vi "DIM_DIO.get service names.vi"(0 "i ref in":refnum<vi>, 5 "error in (no error)":errorcluster) -> (14 "i ref out":refnum<vi>, 16 "writeService":string, 17 "readService":string, 19 "error out":errorcluster)   [LabVIEW 2014, in "DIM_DIO.lvlib"]
doc: "Gets the names of DIM services that are connected to the digital input and output. If a services name equals \"N/A\", the service does not exist and is not created/connected.\n\nLicense Agreement for this software:\n\nCopyright (C)\nGesellschaft für Schwerionenforschung, GSI\nPlanckstr. 1\n64291 Darmstadt\nGermany\n\nContact: D.Beck@gsi.de \n\nThis program is free software; you can redistribute it and/or modify it under the terms of the GNU General Public License as published by the Free Software Foundation; either version 2 of the license, or (at your option) any later version.\n\nThis program is distributed in the hope that it will be useful, but WITHOUT ANY WARRANTY; without even the implied warranty of MERCHANTABILITY or FITNESS FOR A PARTICULAR PURPOSE. See the GNU General License for more details (http://www.gnu.org).\n\nGesellschaft für Schwerionenforschung, GSI\nPlanckstr. 1, 64291 Darmstadt, Germany\nFor all questions and ideas contact: M.Richter@gsi.de, H.Brand@gsi.de or D.Beck@gsi.de.\nLast update: 17-JUN-2004"
uses:
  DIM_DIO.lvlib
  CSCore/BaseProcess/BaseProcess.lvlib
  CSCore/CSSystem/CSSystemLib/CSSystemLib.lvlib
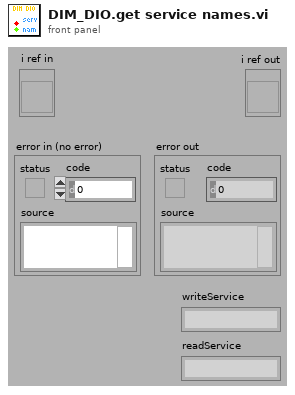
[diagram p1: front panel]
types:
  T1 = typedef "BaseProcess.lvlib/BaseProcess.i attribute.ctl" = cluster{"EventStatus":string, "EventError":i32, "PresetEvtWatchD":i32, "PresetPdcWatchD":i32, "EventTimeout":i32, "PeriodicInterval":i32, "Interface":string[], "Address":string[], "Special":string[], "PeriodicError":i32, "PeriodicStatus":string, "SuperProc":string, "Descriptors":T2[], "CaseRef":refnum<vi>, "PdcRef":refnum<vi>, "Thread Ref":refnum<vi>, "eventErrorID":i32, "eventStatusID":i32, "periodicErrorID":i32, "periodicStatusID":i32, "pdcCtrID":i32}
  T2 = typedef "BaseProcess.lvlib/BaseProcess.descriptor definition.ctl" = cluster{"selector":string, "descriptor":T3}
  T3 = typedef "BaseProcess.lvlib/BaseProcess.descriptor string definition.ctl" = string
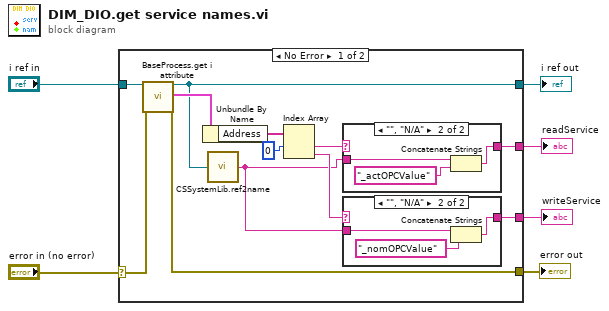
[diagram p0: block diagram]
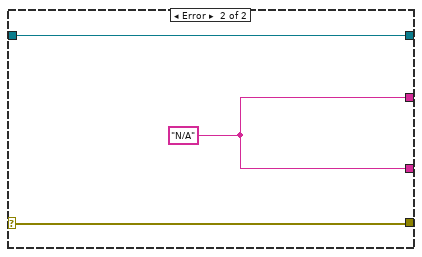
[diagram p4: hidden frame]
diagram:
  n1 = case shown="No Error" "error in (no error)" {
    selector: "error in (no error)" -> [w16 w28]
    tunnel: "i ref in" -> [w18 w29]
    tunnel: [w8 w29] -> w5
    tunnel: [w17 w28] -> w4
    tunnel: [w11 w27] -> w2
    tunnel: [w9 w27] -> w1
    frame No Error {
      n2 = call "BaseProcess.get i attribute.vi"("i ref in"=w18, "error in (no error)"=w16) -> ("i ref out"=w8:refnum<vi>, "i attribute"=w15:T1, "error out"=w17:errorcluster)  [unwired: 15 in]
      n3 = Unbundle By Name(w15) -> ("Address"=w14:string[])
      n4 = call "CSSystemLib.ref2name.vi"("obj refnum"=w8) -> ("name"=w7:string)
      n5 = Index Array(array=w14, index #1=0 ("index")) -> (element #1=w12:string, element #2=w10:string)  [unwired: 1 in]
      n6 = case shown="\"\", \"N/A\"" w12 {
        selector: w12 -> [w23 _]
        tunnel: [w23 w24] -> w11
        tunnel: w7 -> [_ w26]
        frame Default {
        }
        frame "", "N/A" {
          n7 = Concatenate Strings(w26, "_actOPCValue" ("string")) -> (w24:string)
        }
      }
      n8 = case shown="\"\", \"N/A\"" w10 {
        selector: w10 -> [w19 _]
        tunnel: [w19 w20] -> w9
        tunnel: w7 -> [_ w22]
        frame Default {
        }
        frame "", "N/A" {
          n9 = Concatenate Strings(w22, "_nomOPCValue" ("string")) -> (w20:string)
        }
      }
    }
    frame Error {
      w27 = "N/A"
    }
  }
  "error out" <- w4
  "i ref out" <- w5
  "writeService" <- w1
  "readService" <- w2
